vi "EPS-Configure Operation Mode.vi"(8 "error in":errorcluster, 9 "Values":dbl format="%#.3g", 10 "Operation Mode":T1, 11 "EPS Setting In":T2) -> (0 "error out":errorcluster, 3 "EPS Setting Out":T2)   [LabVIEW 2018]
uses:
  Data Def/EPS-Setting.ctl
  Data Def/EPS-Value Type.ctl
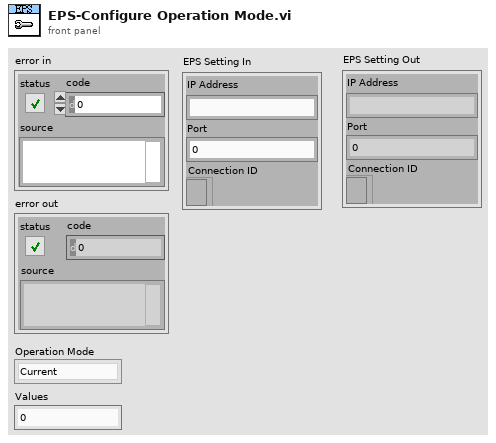
[diagram p1: front panel]
types:
  T1 = typedef "EPS-Value Type.ctl" = enum16{"Current", "Vlotage", "Power"}
  T2 = typedef "EPS-Setting.ctl" = cluster{"IP Address":string, "Port":u16, "Connection ID":refnum<k5>}
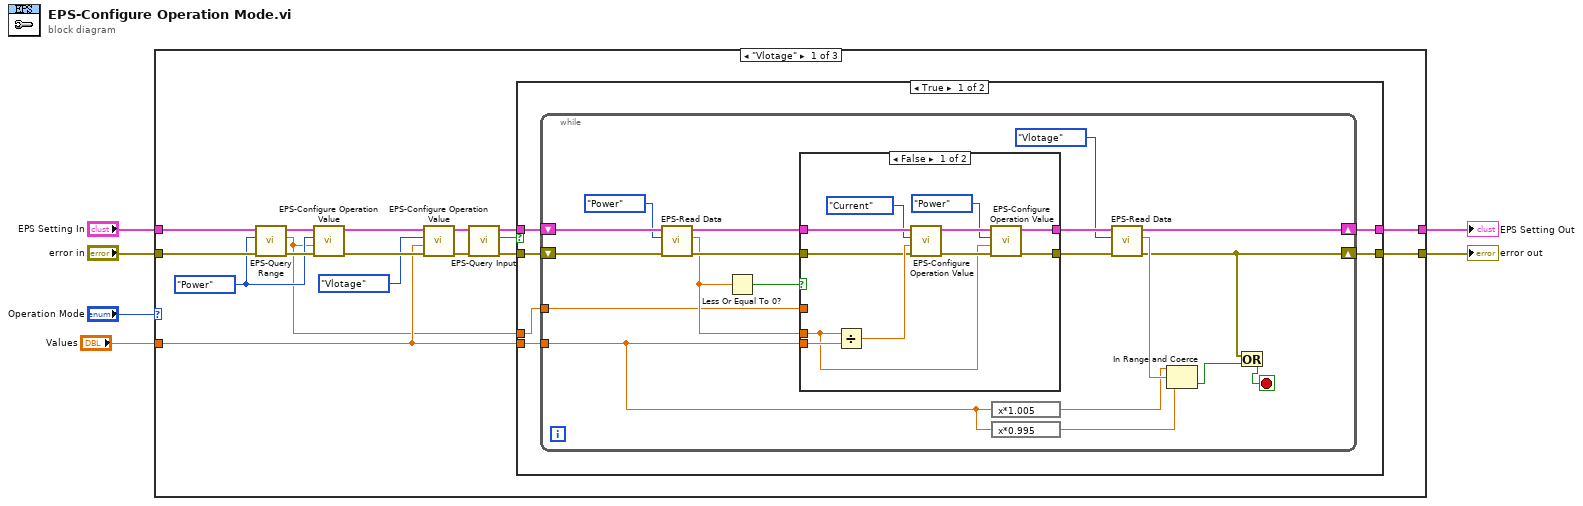
[diagram p0: block diagram]
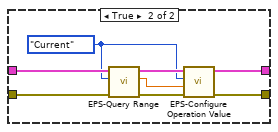
[diagram p2: hidden frame]
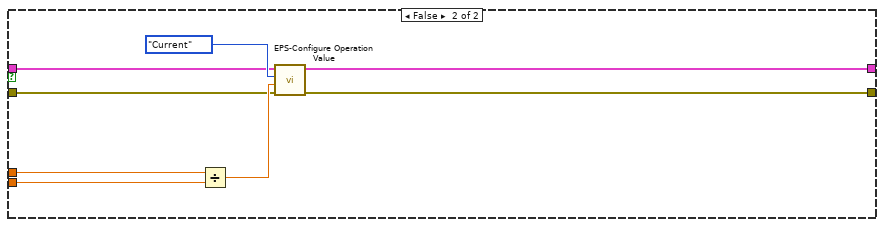
[diagram p3: hidden frame]
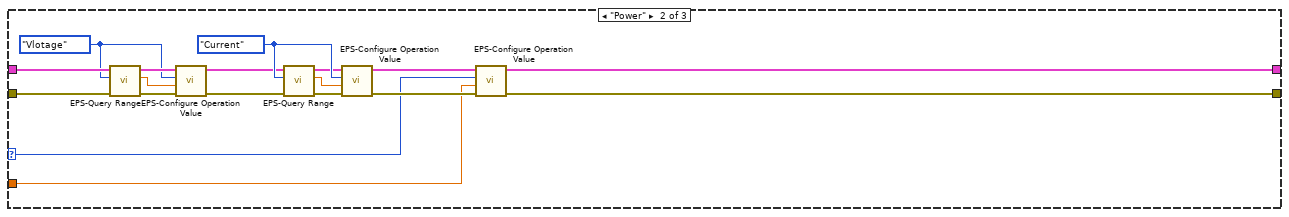
[diagram p4: hidden frame]
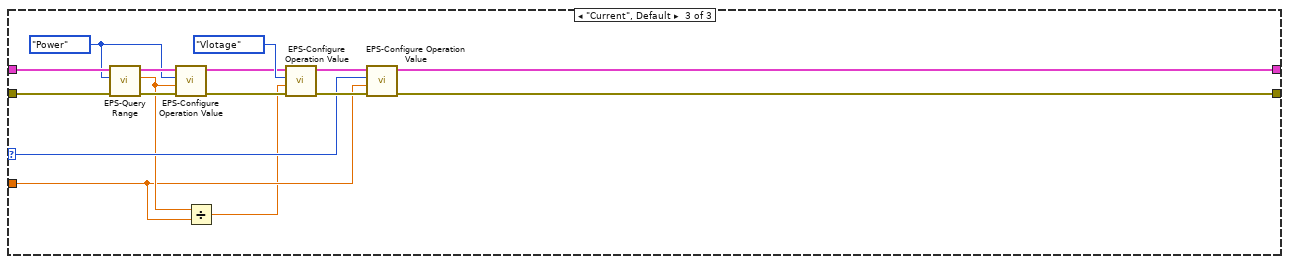
[diagram p5: hidden frame]
diagram:
  n1 = case shown="\"Vlotage\"" "Operation Mode" {
    selector: "Operation Mode" -> [_ w79 w101]
    tunnel: "error in" -> [w23 w93 w109]
    tunnel: "EPS Setting In" -> [w22 w92 w108]
    tunnel: "Values" -> [w10 w78 w95]
    tunnel: [w9 w77 w100] -> w1
    tunnel: [w8 w76 w99] -> w2
    frame "Vlotage" {
      w19 = EPS-Value_Type."Power" ("Value Type")
      n2 = call "EPS-Query Range.vi"("error in"=w23, "Value Type"=w19, "EPS Setting In"=w22) -> ("error out"=w21:errorcluster, "Range"=w7:dbl, "EPS Setting Out"=w20:T2)  [unwired: 6 in]
      n3 = call "EPS-Configure Operation Value.vi"("error in"=w21, "Values"=w7, "Value Type"=w19, "EPS Setting In"=w20) -> ("error out"=w18:errorcluster, "EPS Setting Out"=w17:T2)  [unwired: 6 in]
      n4 = call "EPS-Configure Operation Value.vi"("error in"=w18, "Values"=w10, "Value Type"=EPS-Value_Type."Vlotage", "EPS Setting In"=w17) -> ("error out"=w14:errorcluster, "EPS Setting Out"=w15:T2)  [unwired: 6 in]
      n5 = call "EPS-Query Input.vi"("error in"=w14, "EPS Setting In"=w15) -> ("error out"=w11:errorcluster, "Input?"=w13:bool, "EPS Setting Out"=w12:T2)  [unwired: 7 in]
      n6 = case shown="True" w13 {
        tunnel: w12 -> [w28 w70]
        tunnel: w11 -> [w29 w68]
        tunnel: w10 -> [w27 w75]
        tunnel: [w25 w72] -> w9
        tunnel: [w26 w71] -> w8
        tunnel: w7 -> [w24 w69]
        frame True {
          n7 = while {
            tunnel: w27 -> [w34]
            tunnel: w24 -> [w41]
            shift-right: [w31] -> w25
            shift-left: w29 -> [w48]
            shift-right: [w38] -> w26
            shift-left: w28 -> [w47]
            stop <- w30 stop-if-true
            n8 = call "EPS-Read Data.vi"("error in"=w48, "Value Type"=EPS-Value_Type."Power", "EPS Setting In"=w47) -> ("error out"=w44:errorcluster, "Value"=w43:dbl, "EPS Setting Out"=w45:T2)  [unwired: 6 in]
            n9 = Less Or Equal To 0?(x=w43) -> (x <= 0?=w42:bool)
            n10 = case shown="False" w42 {
              tunnel: w34 -> [w59 _]
              tunnel: w45 -> [w58 w67]
              tunnel: w44 -> [w55 w66]
              tunnel: [w53 w60] -> w39
              tunnel: [w51 w61] -> w40
              tunnel: w43 -> [w49 _]
              tunnel: w41 -> [_ _]
              frame False {
                n11 = Divide(x=w49, y=w59) -> (x/y=w57:dbl)
                n12 = call "EPS-Configure Operation Value.vi"("error in"=w55, "Values"=w57, "Value Type"=EPS-Value_Type."Current", "EPS Setting In"=w58) -> ("error out"=w52:errorcluster, "EPS Setting Out"=w54:T2)  [unwired: 6 in]
                n13 = call "EPS-Configure Operation Value.vi"("error in"=w52, "Values"=w49, "Value Type"=EPS-Value_Type."Power", "EPS Setting In"=w54) -> ("error out"=w51:errorcluster, "EPS Setting Out"=w53:T2)  [unwired: 6 in]
              }
              frame True {
                w62 = EPS-Value_Type."Current" ("Value Type")
                n14 = call "EPS-Query Range.vi"("error in"=w66, "Value Type"=w62, "EPS Setting In"=w67) -> ("error out"=w64:errorcluster, "Range"=w63:dbl, "EPS Setting Out"=w65:T2)  [unwired: 6 in]
                n15 = call "EPS-Configure Operation Value.vi"("error in"=w64, "Values"=w63, "Value Type"=w62, "EPS Setting In"=w65) -> ("error out"=w61:errorcluster, "EPS Setting Out"=w60:T2)  [unwired: 6 in]
              }
            }
            n16 = expression code="x*1.005"(w34) -> (w35:dbl)
            n17 = expression code="x*0.995"(w34) -> (w33:dbl)
            n18 = call "EPS-Read Data.vi"("error in"=w40, "Value Type"=EPS-Value_Type."Vlotage", "EPS Setting In"=w39) -> ("error out"=w31:errorcluster, "Value"=w36:dbl, "EPS Setting Out"=w38:T2)  [unwired: 6 in]
            n19 = In Range and Coerce(upper limit=w35, x=w36, lower limit=w33) -> (In Range?=w32:bool)  [unwired: 1 out]
            n20 = Or(x=w31, y=w32) -> (x .or. y?=w30:bool)
          }
        }
        frame False {
          n21 = Divide(x=w69, y=w75) -> (x/y=w74:dbl)
          n22 = call "EPS-Configure Operation Value.vi"("error in"=w68, "Values"=w74, "Value Type"=EPS-Value_Type."Current", "EPS Setting In"=w70) -> ("error out"=w72:errorcluster, "EPS Setting Out"=w71:T2)  [unwired: 6 in]
        }
      }
    }
    frame "Power" {
      w87 = EPS-Value_Type."Current" ("Value Type")
      w88 = EPS-Value_Type."Vlotage" ("Value Type")
      n23 = call "EPS-Query Range.vi"("error in"=w93, "Value Type"=w88, "EPS Setting In"=w92) -> ("error out"=w91:errorcluster, "Range"=w90:dbl, "EPS Setting Out"=w89:T2)  [unwired: 6 in]
      n24 = call "EPS-Configure Operation Value.vi"("error in"=w91, "Values"=w90, "Value Type"=w88, "EPS Setting In"=w89) -> ("error out"=w83:errorcluster, "EPS Setting Out"=w82:T2)  [unwired: 6 in]
      n25 = call "EPS-Query Range.vi"("error in"=w83, "Value Type"=w87, "EPS Setting In"=w82) -> ("error out"=w84:errorcluster, "Range"=w85:dbl, "EPS Setting Out"=w86:T2)  [unwired: 6 in]
      n26 = call "EPS-Configure Operation Value.vi"("error in"=w84, "Values"=w85, "Value Type"=w87, "EPS Setting In"=w86) -> ("error out"=w81:errorcluster, "EPS Setting Out"=w80:T2)  [unwired: 6 in]
      n27 = call "EPS-Configure Operation Value.vi"("error in"=w81, "Values"=w78, "Value Type"=w79, "EPS Setting In"=w80) -> ("error out"=w77:errorcluster, "EPS Setting Out"=w76:T2)  [unwired: 6 in]
    }
    frame "Current", Default {
      w105 = EPS-Value_Type."Power" ("Value Type")
      n28 = call "EPS-Query Range.vi"("error in"=w109, "Value Type"=w105, "EPS Setting In"=w108) -> ("error out"=w107:errorcluster, "Range"=w96:dbl, "EPS Setting Out"=w106:T2)  [unwired: 6 in]
      n29 = call "EPS-Configure Operation Value.vi"("error in"=w107, "Values"=w96, "Value Type"=w105, "EPS Setting In"=w106) -> ("error out"=w97:errorcluster, "EPS Setting Out"=w98:T2)  [unwired: 6 in]
      n30 = Divide(x=w96, y=w95) -> (x/y=w94:dbl)
      n31 = call "EPS-Configure Operation Value.vi"("error in"=w97, "Values"=w94, "Value Type"=EPS-Value_Type."Vlotage", "EPS Setting In"=w98) -> ("error out"=w103:errorcluster, "EPS Setting Out"=w102:T2)  [unwired: 6 in]
      n32 = call "EPS-Configure Operation Value.vi"("error in"=w103, "Values"=w95, "Value Type"=w101, "EPS Setting In"=w102) -> ("error out"=w100:errorcluster, "EPS Setting Out"=w99:T2)  [unwired: 6 in]
    }
  }
  "error out" <- w1
  "EPS Setting Out" <- w2
